vi "fft.vi"() -> ()   [LabVIEW 2023]
uses:
  Images/_Images.ctl
  <vilib>/vision/NI_Vision_Development_Module.lvlib
panel:
  in  "Image 3":T1
  out "Image 2":T2(plugin-control)
  out "Image":T2(plugin-control)
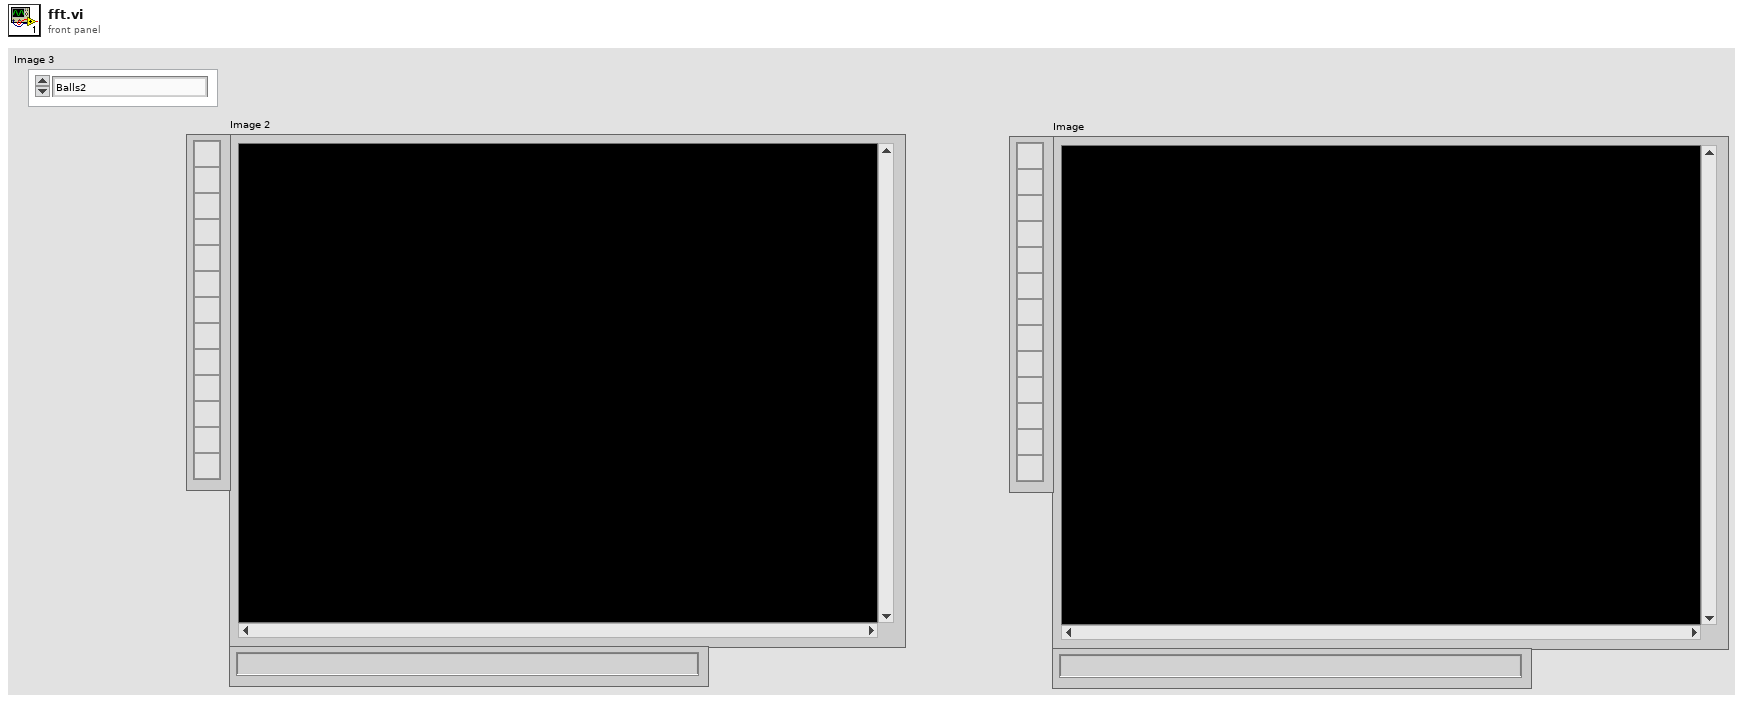
[diagram p1: front panel]
types:
  T1 = typedef "_Images.ctl" = enum16{"Balls2", "Battery1", "Battery2", "Connector1", "Subwoofer1", "Subwoofer2", "Subwoofer3", "Subwoofer4", "Hase1", "Lamp1", "Lamp2", "Mouse1", "PhotoLens1", "Po1", "PowerSupply1", "Router", "--- Step Wedges ---", "Stepwedge1", "Stepwedge2", "Stepwedge3", "--- Fusion ---", "Fusion160kV", "Fusion2-120kV", "Fusion2-320kV", "Fusion300kV", "FusionPart1-120kV", "FusionPart1-180kV", "--- PART 01 ---", "Part1", "Part2", "Part3", "Part4", "Part5", "Part6", "Part7", "Part8", "--- Different Integrations ---", "Step2737-02Int", "Step2737-04Int", "Step2737-08Int", "Step2737-16Int", "Step2737-32Int", "Step2737-64Int"}
  T2 = typedef "IMAQ Image.ctl" = refnum<image>
  T3 = typedef "Image Type" = u32
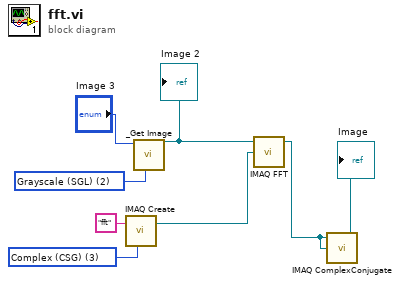
[diagram p0: block diagram]
diagram:
  w4 = T3 3 items=["Grayscale (U8)", "Grayscale (I16)", "Grayscale (SGL)", "Complex (CSG)", "RGB (U32)", "HSL (U32)", "RGB (U64)", "Grayscale (U16)"] ("Image Type")
  w8 = T3 2 items=["Grayscale (U8)", "Grayscale (I16)", "Grayscale (SGL)", "Complex (CSG)", "RGB (U32)", "HSL (U32)", "RGB (U64)", "Grayscale (U16)"] ("Image Type (U16)")
  n1 = call "IMAQ Create"("Image Name"="fft", "Image Type"=w4) -> ("New Image"=w5:T2)  [unwired: 3 in, 1 out]
  n2 = call "_Get Image.vi"("Image Type (U16)"=w8, "Image"="Image 3") -> ("Image Out"=w3:T2)  [unwired: 6 in, 3 out]
  "Image 2" <- w3
  n3 = call "IMAQ FFT"("Image Dst"=w5, "Image Src"=w3) -> ("Image Dst Out"=w1:T2)  [unwired: 2 in, 1 out]
  n4 = call "IMAQ ComplexConjugate"("Image Dst"=w1, "Image Src"=w1) -> ("Image Dst Out"=→"Image":T2)  [unwired: 2 in, 1 out]
